vi "Main.vi"() -> ()   [LabVIEW 2013]
uses:
  Globals.vi
panel:
  in  "Update Global":bool
  out "Global Slide Value":dbl(slide) scale=0.0..10.0
  in  "Slide":dbl(slide) scale=0.0..10.0
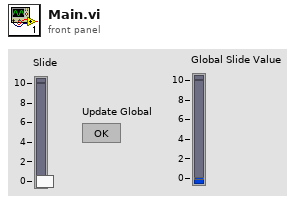
[diagram p1: front panel]
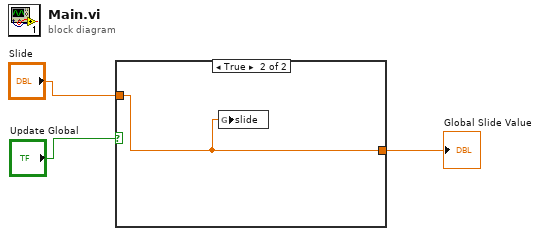
[diagram p0: block diagram]
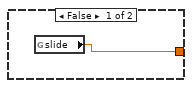
[diagram p2: hidden frame]
diagram:
  n1 = case shown="True" "Update Global" {
    tunnel: "Slide" -> [_ w5]
    tunnel: [w4 w5] -> w1
    frame False {
      n2 = global read "Globals.vi" "slide"() -> (w4:dbl)
    }
    frame True {
      n3 = global write "Globals.vi" "slide"(w5) -> ()
    }
  }
  "Global Slide Value" <- w1
